vi "Create Box.vi"(7 "Color":T1={"Red"=1.0, "Green"=0.0, "Blue"=0.0, "Alpha"=1.0}, 8 "error in (no error)":errorcluster, 9 "Length Z":sgl=1.0, 10 "Length Y":sgl=1.0, 11 "Length X":sgl=1.0) -> (0 "error out":errorcluster, 3 "New Box Refnum":refnum<vi>)   [LabVIEW 2020, in "NI_3D Picture Control.lvlib"]
doc: "Sets a 3D object you create with the Create Object VI to a box by applying a box geometry to the object."
uses:
  NI_3D Picture Control.lvlib
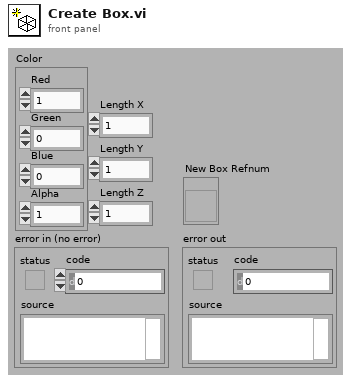
[diagram p1: front panel]
types:
  T1 = cluster{"Red":sgl, "Green":sgl, "Blue":sgl, "Alpha":sgl}
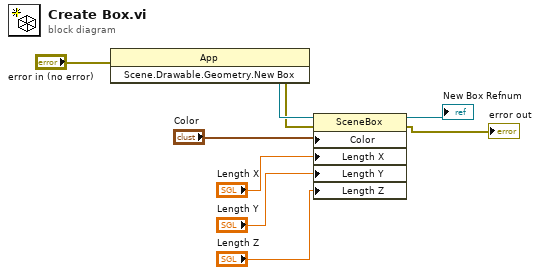
[diagram p0: block diagram]
diagram:
  n1 = invoke class="App" method="Scene.Drawable.Geometry.New Box"(error in="error in (no error)") -> (error out=w3:errorcluster, "Scene.Geometry.New Box"=w9:refnum<vi>)  [unwired: 2 in, 1 out]
  n2 = property class="SceneBox"(reference=w9, error in=w3, "Color"="Color", "Length X"="Length X", "Length Y"="Length Y", "Length Z"="Length Z") -> (reference out=→"New Box Refnum":refnum<vi>, error out=→"error out":errorcluster)
